vi "subSoftinfo.vi"() -> ()   [LabVIEW 2020]
panel:
  in  "Close":bool
  # "PS 35, Version 2.01"
  # "Staufen, Germany"
  # "Copyright (C) by"
  # "OWIS GmbH"
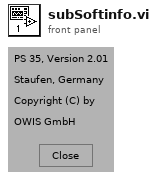
[diagram p1: front panel]
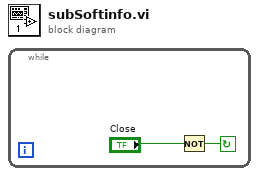
[diagram p0: block diagram]
diagram:
  n1 = while {
    stop <- w2 continue-if-true
    n2 = Not(x="Close") -> (.not. x?=w2:bool)
  }
